vi "Module-Add.vi"(8 "error in":errorcluster, 11 "UUT":T1={"Name"="1", "FrameColor"=16860, "TextColor"=46135, "BGColor"=16777216, "LibBackColor"=16860, "LibTextColor"=16448250, "LibTextSize"=10, "LibTextFont"="Arial", "LibTextBold"=FALSE}) -> (0 "error out":errorcluster)   [LabVIEW 2015, in "Settings-Style.lvlib"]
uses:
  Settings-Style.lvlib
  1_ctl/btn-ok.ctl
  1_ctl/btn-cancel.ctl
  1_Ctl/DB_UUT.ctl
  1_ctl/Ctl-Color.ctl
  1_Ctl/DB_Add_StateMach.ctl
panel:
  in  "Save Name":string
  in  "Cancel":T3
  in  "Save":T4
  # "Style Settings"
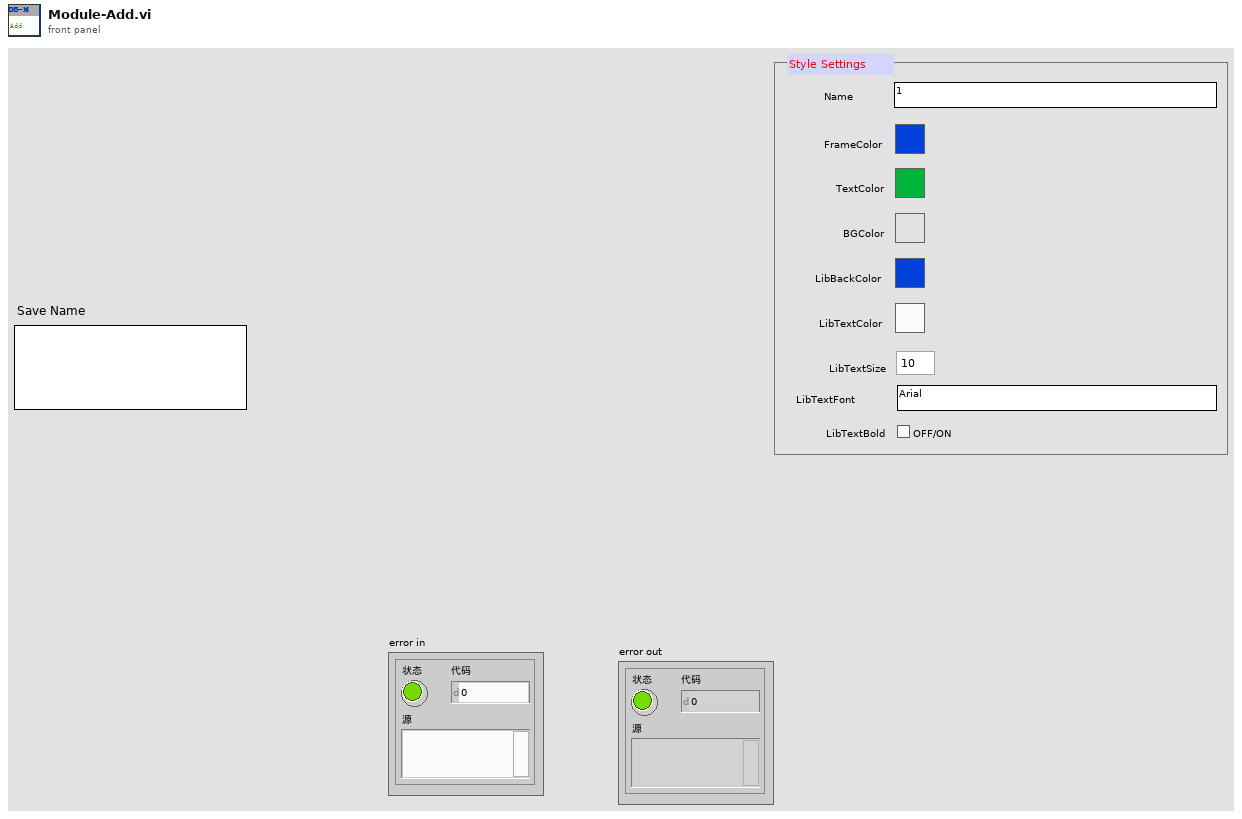
[diagram p1: front panel]
types:
  T1 = typedef "Settings-Style.lvlib/DB_UUT.ctl" = cluster{"Name":string, "FrameColor":T2, "TextColor":T2, "BGColor":T2, "LibBackColor":T2, "LibTextColor":T2, "LibTextSize":u32, "LibTextFont":string, "LibTextBold":bool}
  T2 = typedef "Ctl-Color.ctl" = u32
  T3 = typedef "btn-cancel.ctl" = bool
  T4 = typedef "btn-ok.ctl" = bool
  T5 = typedef "Settings-Style.lvlib/DB_Add_StateMach.ctl" = enum16{"Initialize", "Add--Begin", "Add--Done", "Check_Name_Exist?", "Idle", "Error", "WrongState", "Cancel", "SaveData", "Stop"}
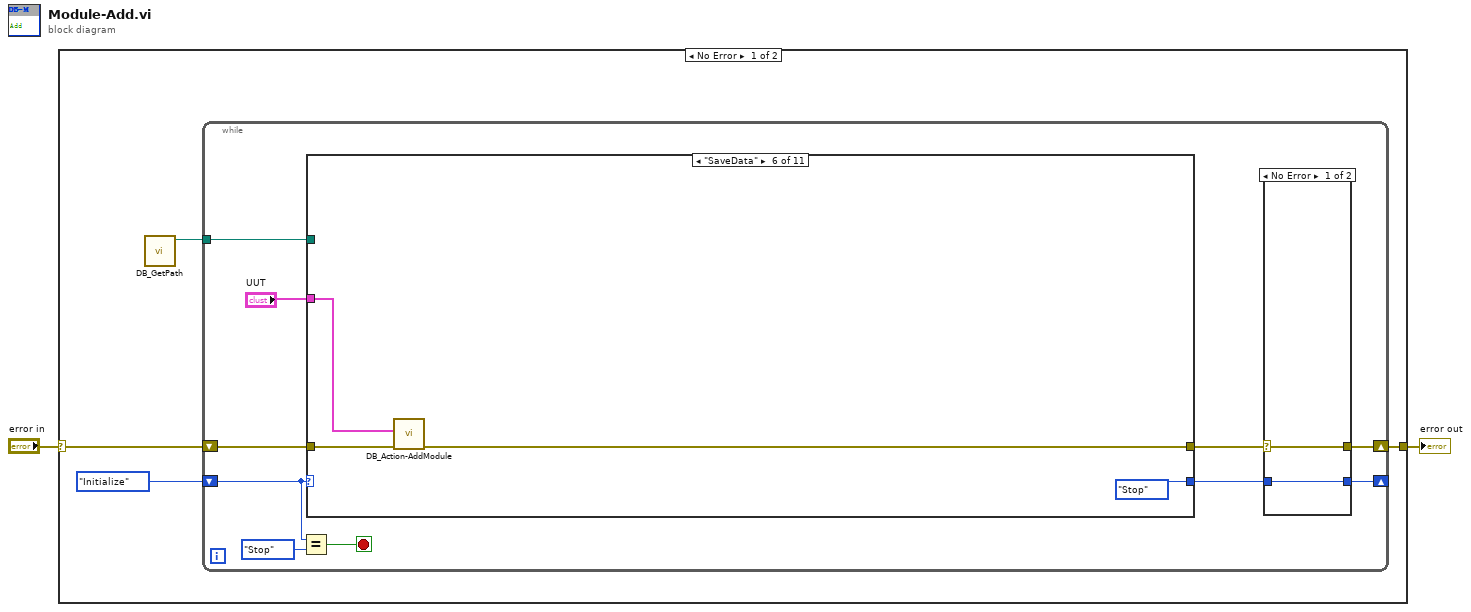
[diagram p0: block diagram]
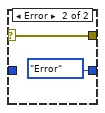
[diagram p2: hidden frame]
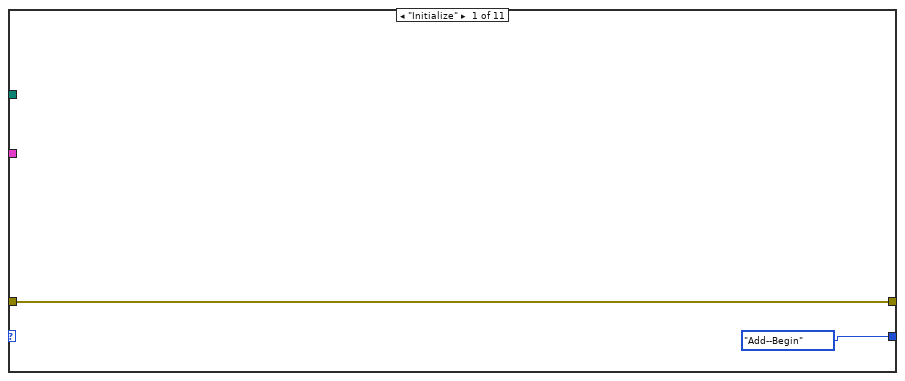
[diagram p3: hidden frame]
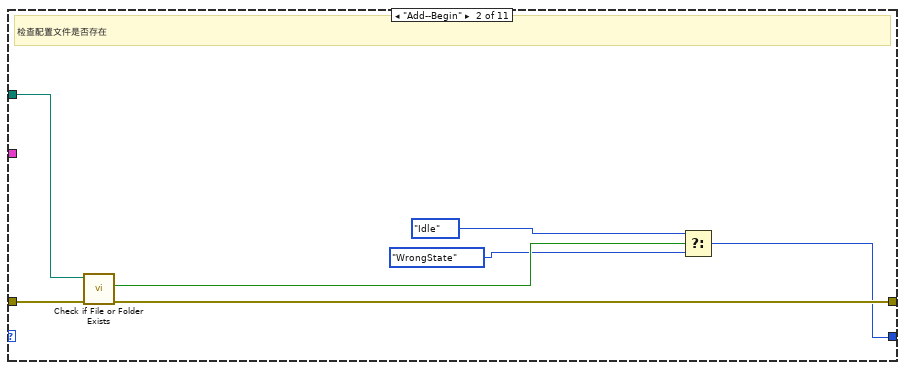
[diagram p4: hidden frame]
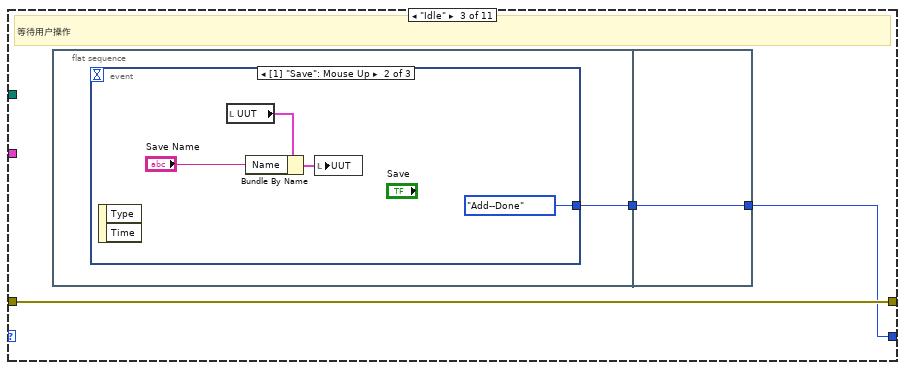
[diagram p5: hidden frame]
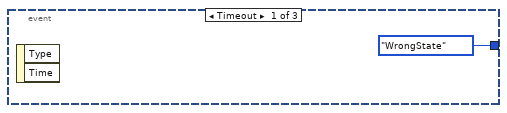
[diagram p6: hidden frame]
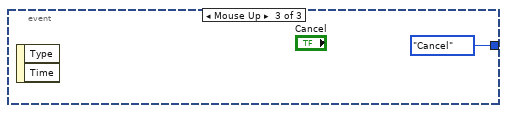
[diagram p7: hidden frame]
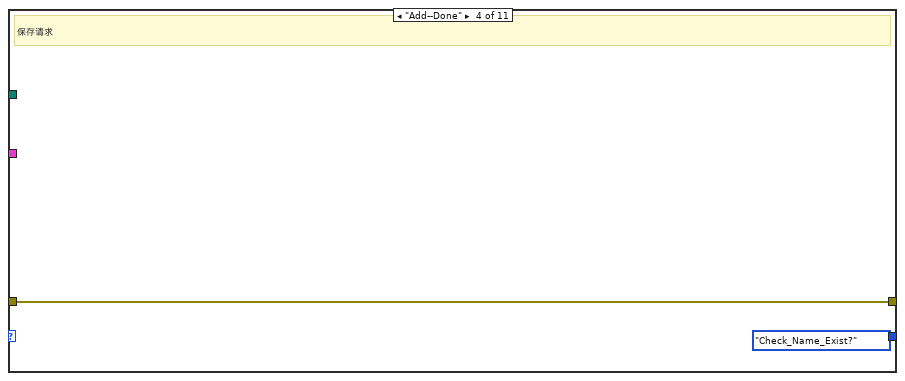
[diagram p8: hidden frame]
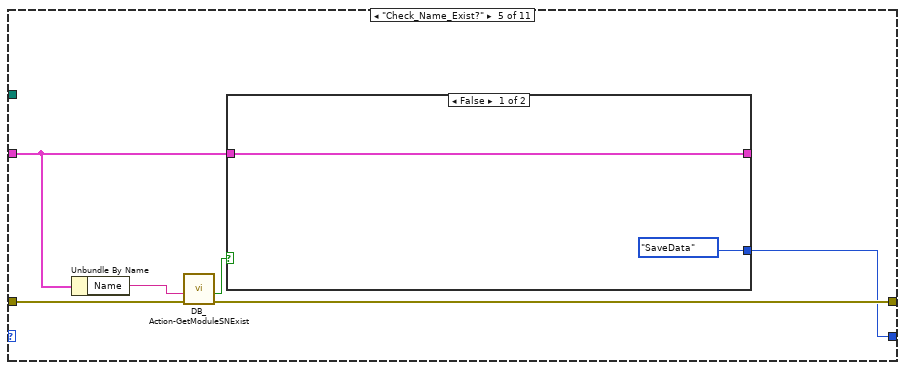
[diagram p9: hidden frame]
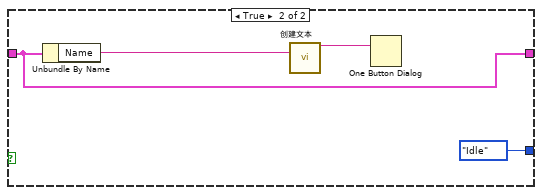
[diagram p10: hidden frame]
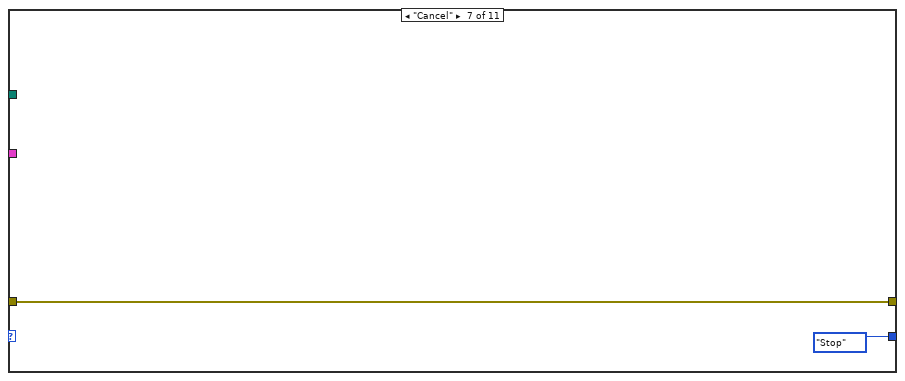
[diagram p11: hidden frame]
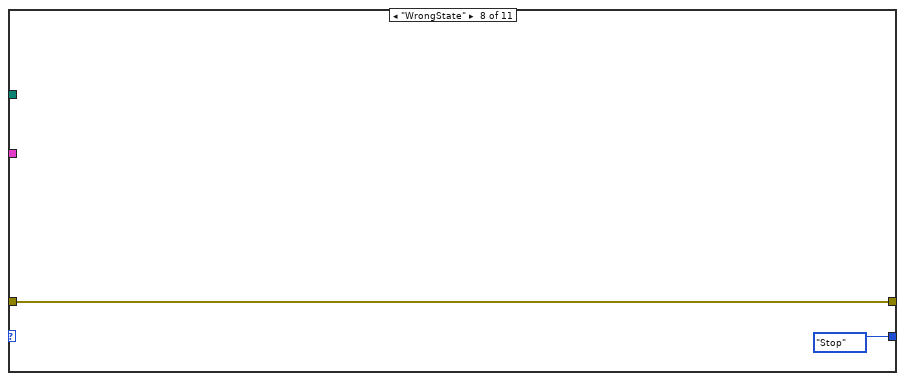
[diagram p12: hidden frame]
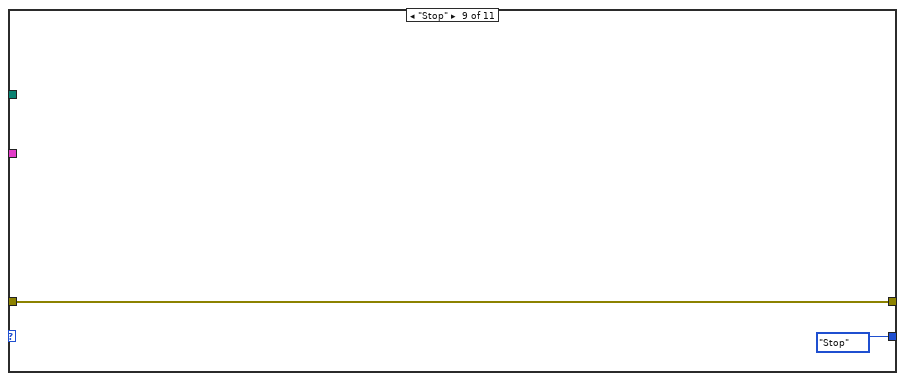
[diagram p13: hidden frame]
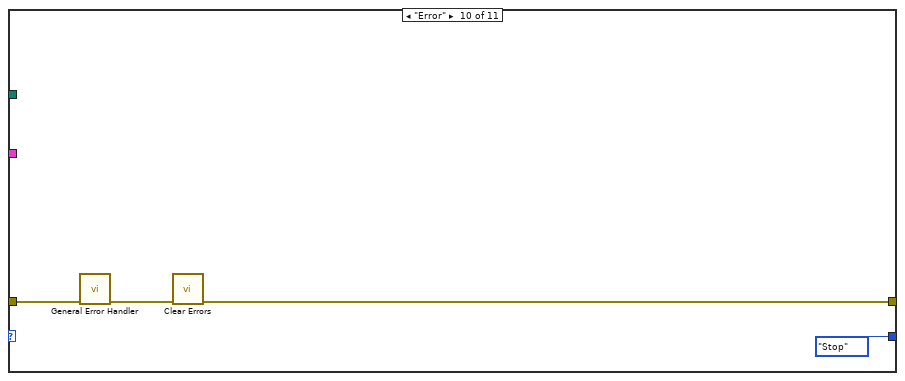
[diagram p14: hidden frame]
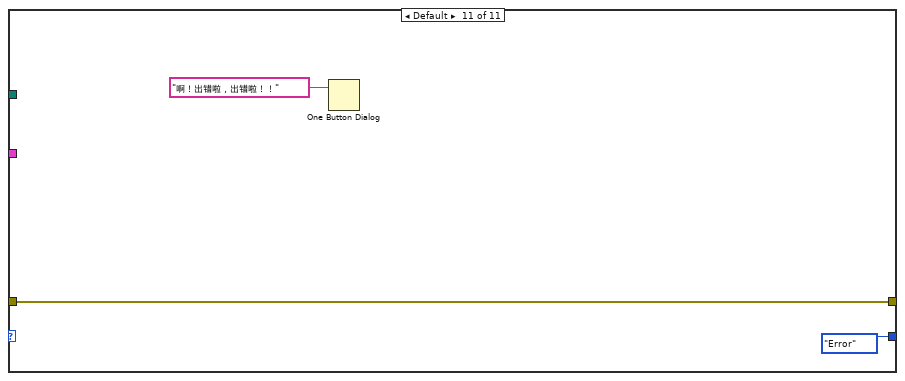
[diagram p15: hidden frame]
diagram:
  n1 = case shown="No Error" "error in" {
    selector: "error in" -> [w5 w72]
    tunnel: [w6 w72] -> w2
    frame No Error {
      n2 = call "DB_GetPath.vi"() -> ("appended path"=w3:path)  [unwired: 11 in]
      n3 = while {
        shift-right: [w10] -> _
        shift-left: DB_Add_StateMach."Initialize" ("Beginning State") -> [w11]
        shift-right: [w12] -> w6
        shift-left: w5 -> [w14]
        tunnel: w3 -> [w8]
        stop <- w16 stop-if-true
        n4 = Equal?(x=w11, y=DB_Add_StateMach."Stop" ("Beginning State")) -> (x = y?=w16:bool)
        n5 = case shown="\"SaveData\"" w11 {
          tunnel: "UUT" -> [_ _ _ _ w44 w56 _ _ _ _ _]
          tunnel: w14 -> [w22 w28 w32 w42 w48 w57 w60 w62 w64 w68 w70]
          tunnel: [w22 w27 w32 w42 w47 w55 w60 w62 w64 w66 w70] -> w13
          tunnel: w8 -> [_ w29 _ _ _ _ _ _ _ _ _]
          tunnel: [DB_Add_StateMach."Add--Begin" ("Beginning State") w23 w31 DB_Add_StateMach."Check_Name_Exist?" ("Beginning State") w46 DB_Add_StateMach."Stop" ("Beginning State") DB_Add_StateMach."Stop" ("Beginning State") DB_Add_StateMach."Stop" ("Beginning State") DB_Add_StateMach."Stop" ("Beginning State") DB_Add_StateMach."Stop" ("Beginning State") DB_Add_StateMach."Error" ("Beginning State")] -> w9
          frame "Initialize" {
          }
          frame "Add--Begin" {
            # "检查配置文件是否存在"
            n6 = call <vilib>:"Check if File or Folder Exists.vi"("error in (no error)"=w28, "path"=w29) -> ("error out"=w27:errorcluster, "file or folder exists?"=w26:bool)  [unwired: 7 in, 1 out]
            n7 = Select(t=DB_Add_StateMach."Idle" ("Beginning State"), s=w26, f=DB_Add_StateMach."WrongState" ("Beginning State")) -> (s? t:f=w23:T5)
          }
          frame "Idle" {
            # "等待用户操作"
            n8 = flat-sequence {
              tunnel: [w33] -> w30
              tunnel: [w40] -> w31
              tunnel: w30 -> [w40]
              frame #0 {
                n9 = event shown="[1] \"Save\": Mouse Up" {
                  selector: _ -> [_ _ _]
                  dyn-events: _ -> [_ _ _]
                  timeout: _ -> [_ _ _]
                  tunnel: [DB_Add_StateMach."WrongState" ("Beginning State") DB_Add_StateMach."Add--Done" ("Beginning State") DB_Add_StateMach."Cancel" ("Beginning State")] -> w33
                  event Timeout {
                    n10 = event-data() -> ()  [unwired: 1 in, 2 out]
                  }
                  event Mouse Up {
                    n11 = event-data() -> ()  [unwired: 1 in, 2 out]
                    n12 = local read "UUT"() -> (w37:T1)
                    n13 = Bundle By Name(cluster=w37, "Name"="Save Name") -> (w35:T1)
                    n14 = local write "UUT"(w35) -> ()
                  }
                  event Mouse Up {
                    n15 = event-data() -> ()  [unwired: 1 in, 2 out]
                  }
                }
              }
              frame #1 {
              }
            }
          }
          frame "Add--Done" {
            # "保存请求"
          }
          frame "Check_Name_Exist?" {
            n16 = Unbundle By Name(w44) -> ("Name"=w43:string)
            n17 = call "DB_Action-GetModuleSNExist.vi"("error in"=w48, "Name"=w43) -> ("error out"=w47:errorcluster, "ID_Exist?"=w45:bool)  [unwired: 8 in]
            n18 = case shown="False" w45 {
              tunnel: [DB_Add_StateMach."SaveData" ("Beginning State") DB_Add_StateMach."Idle" ("Beginning State")] -> w46
              tunnel: w44 -> [w49 w53]
              tunnel: [w49 w53] -> _
              frame False {
              }
              frame True {
                n19 = Unbundle By Name(w53) -> ("Name"=w51:string)
                n20 = call "创建文本"("Name"=w51) -> ("Result"=w52:string)  [unwired: 13 in, 1 out]
                n21 = One Button Dialog(message=w52) -> ()  [unwired: 1 in, 1 out]
              }
            }
          }
          frame "SaveData" {
            n22 = call "DB_Action-AddModule.vi"("error in"=w57, "UUT输入"=w56) -> ("error out"=w55:errorcluster)  [unwired: 9 in]
          }
          frame "Cancel" {
          }
          frame "WrongState" {
          }
          frame "Stop" {
          }
          frame "Error" {
            n23 = call <vilib>:"General Error Handler.vi"("error in (no error)"=w68) -> ("error out"=w67:errorcluster)  [unwired: 10 in, 4 out]
            n24 = call <vilib>:"Clear Errors.vi"("error in (no error)"=w67) -> ("error out"=w66:errorcluster)  [unwired: 5 in, 1 out]
          }
          frame Default {
            n25 = One Button Dialog(message="啊！出错啦，出错啦！！" ("消息")) -> ()  [unwired: 1 in, 1 out]
          }
        }
        n26 = case shown="No Error" w13 {
          selector: w13 -> [w18 w20]
          tunnel: [w18 w20] -> w12
          tunnel: [w17 DB_Add_StateMach."Error" ("Beginning State")] -> w10
          tunnel: w9 -> [w17 _]
          frame No Error {
          }
          frame Error {
          }
        }
      }
    }
    frame Error {
    }
  }
  "error out" <- w2
